vi "String to Boolean.vi"(8 "error in (no error)":errorcluster, 11 "Boolean String":string) -> (0 "error out":errorcluster, 3 "Boolean":bool)   [LabVIEW 2024]
doc: "Converts a string to a Boolean and generates a user-defined error if the conversion fails."
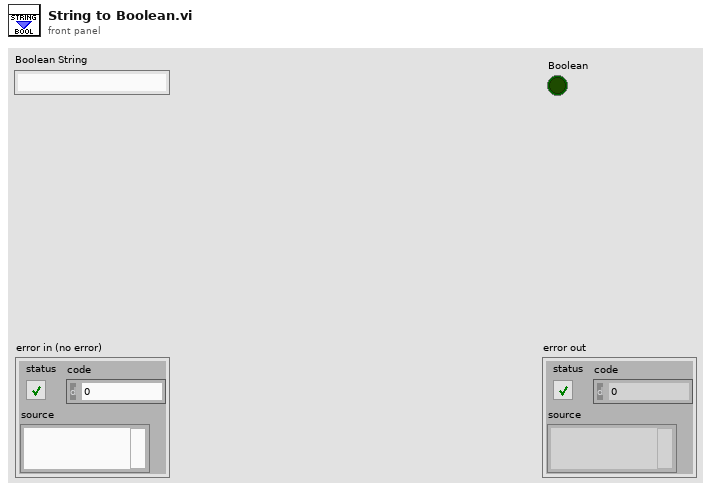
[diagram p1: front panel]
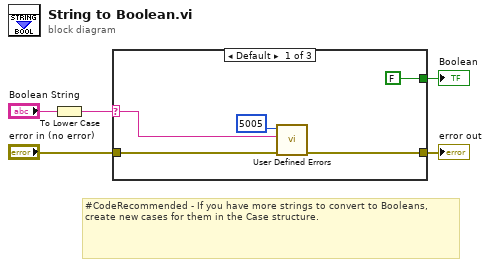
[diagram p0: block diagram]
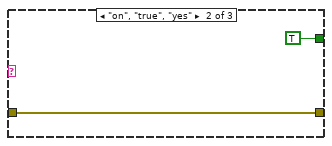
[diagram p2: hidden frame]
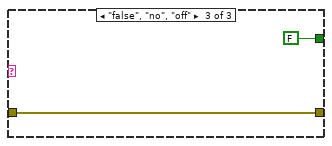
[diagram p3: hidden frame]
diagram:
  # "#CodeRecommended - If you have more strings to convert to Booleans, create new cases for them in the Case structure."
  n1 = To Lower Case(string="Boolean String") -> (all lower case string=w2:string)
  n2 = case shown="Default" w2 {
    selector: w2 -> [w7 _ _]
    tunnel: [w9 w11 w13] -> w4
    tunnel: "error in (no error)" -> [w6 w11 w13]
    tunnel: [FALSE ("Boolean") TRUE ("Boolean") FALSE ("Boolean")] -> w1
    frame Default {
      n3 = call "User Defined Errors.vi"("error in (no error)"=w6, "Parameter 1"=w7, "Error Code (0)"=5005 ("error code (0)")) -> ("error out"=w9:errorcluster)  [unwired: 8 in]
    }
    frame "on", "true", "yes" {
    }
    frame "false", "no", "off" {
    }
  }
  "error out" <- w4
  "Boolean" <- w1
